vi "Inspect.vi"(8 "Error in":errorcluster, 9 "Msg":refnum<class "Msg.lvclass">, 10 "Within Unified Msgs":bool, 11 "TEMPLATE Actor in":refnum<class "TEMPLATE Actor.lvclass">) -> (2 "Proceed":bool=TRUE, 3 "TEMPLATE Actor out":refnum<class "TEMPLATE Actor.lvclass">)   [LabVIEW 2025, in "_Template.lvlib" / "Templates.lvlib" / "TEMPLATE jettl Actor.lvlib" / "TEMPLATE Actor.lvlib" / "TEMPLATE Actor.lvclass"]
uses:
  TEMPLATE Actor.lvclass
  jettl/jettl/Msg/Msg.lvclass
  TEMPLATE Actor.lvclass/TEMPLATE Actor.ctl
  jettl/jettl/jettl.lvlib
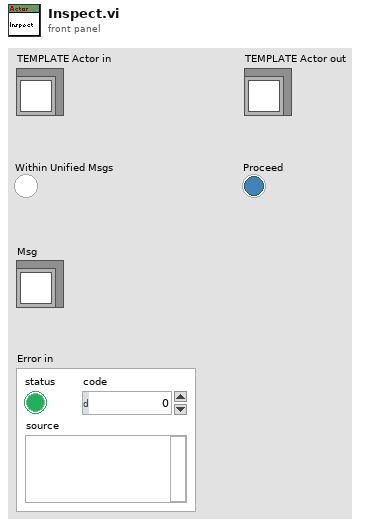
[diagram p1: front panel]
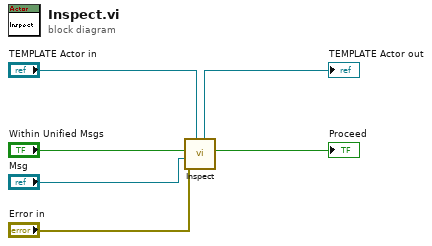
[diagram p0: block diagram]
diagram:
  n1 = call "Inspect.vi"("Actor in"="TEMPLATE Actor in", "Error in"="Error in", "Msg"="Msg", "Within Unified Msgs"="Within Unified Msgs") -> ("Proceed"=→"Proceed":bool, "Actor out"=→"TEMPLATE Actor out":refnum<class "TEMPLATE Actor.lvclass">)  [unwired: 6 in]
